vi "Shooter.vi"(4 "Ball Count":i8=3, 6 "Aquire Fail Action":T1, 7 "Distance":dbl, 8 "error in (no error)":errorcluster, 9 "Use Camera":bool, 10 "Test":bool, 11 "Fire":bool) -> (0 "error out":errorcluster, 3 "Shooter State":T1)   [LabVIEW 2011]
uses:
  ShooterStates.ctl
  Robot Global Data.vi
  <vilib>/Rock Robotics/WPI/Solenoid/Deprecated/WPI_SolenoidSetBool.vi
panel:
  in  "Second Spinup Timeout (ms)":u32=2000
  in  "PostSensor(ms)":u32=50
  in  "First Spinup Timeout (ms)":u32=3000
  out "Shot":bool
  in  "Top Rollers Speed":dbl=-1.0
  in  "Max Shoot Time (ms)":u32=2000
  # "Shoot"
  # "Spinup"
  # "Run Shooter\nOnly"
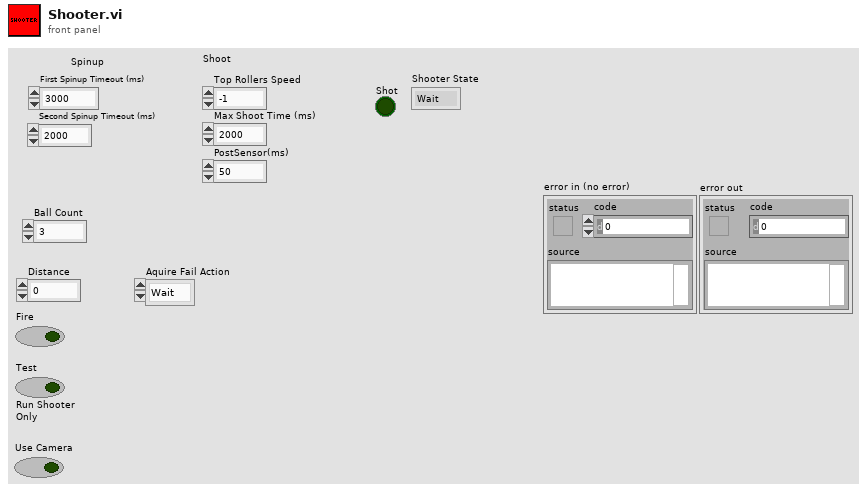
[diagram p1: front panel]
types:
  T1 = typedef "ShooterStates.ctl" = enum16{"Wait", "Aquire", "SpinUp", "Shoot", "Test"}
  T2 = typedef "Semaphore RefNum" = refnum<k1>
  T3 = cluster{"Aquire Target":bool, "Target Aquired":bool, "Attempts":dbl}
  T4 = typedef "ShooterData.ctl" = cluster{"Setpoint":dbl, "Speed":dbl, "Squish":dbl, "Shot Sensor":bool, "At Speed":bool}
  T5 = typedef "WPI_DigitalInputDevRef.ctl" = cluster{"DevStatus":errorcluster, "DIO Channel":T6, "Digital Module":T7}
  T6 = typedef "FPGA_DIOChannel.ctl" = enum8{"DIO 1", "DIO 2", "DIO 3", "DIO 4", "DIO 5", "DIO 6", "DIO 7", "DIO 8", "DIO 9", "DIO 10", "DIO 11", "DIO 12", "DIO 13", "DIO 14", "Invalid"}
  T7 = typedef "FPGA_TypedefDigitalModule.ctl" = enum16{"Digital Module 1", "Digital Module 2"}
  T8 = typedef "WPI_SolenoidDevRef.ctl" = cluster{"DevStatus":errorcluster, "Solenoid Module":T9, "Forward Solenoid Channel":T10, "Reverse Solenoid Channel":T10}
  T9 = typedef "FPGA_TypedefSolenoidModule.ctl" = enum16{"Solenoid Module 1", "Solenoid Module 2"}
  T10 = typedef "WPI_SolenoidChannel.ctl" = enum8{"Solenoid 1", "Solenoid 2", "Solenoid 3", "Solenoid 4", "Solenoid 5", "Solenoid 6", "Solenoid 7", "Solenoid 8", "Invalid"}
  T11 = typedef "WPI_MotorControlDeviceRef.ctl" = cluster{"DeviceStatus":errorcluster, "Type":enum16{"PWM", "CAN"}, "PWM":cluster{"Digital Module":T7, "PWM Channel":T12, "DeadBand":T13}, "CAN":cluster{"Device Number":u8, "Control Mode":T14, "Semaphore":T2, "Max Vout":dbl}, "Invert":bool, "TransformRef":T15, "InvTransformRef":T15}
  T12 = typedef "FPGA_DIOPWMChannel.ctl" = enum8{"PWM 1", "PWM 2", "PWM 3", "PWM 4", "PWM 5", "PWM 6", "PWM 7", "PWM 8", "PWM 9", "PWM 10", "Invalid"}
  T13 = typedef "WPI_PWMDeadband.ctl" = cluster{"Name":string, "maxPositivePwm":i32, "minPositivePwm":i32, "centerPwm":i32, "maxNegativePwm":i32, "minNegativePwm":i32, "angularRange":u16}
  T14 = typedef "WPI_CANJaguar_ControlMode.ctl" = enum8{"Percent VBus", "Current", "Speed", "Position", "Voltage"}
  T15 = typedef "WPI_PWMTransform_ConPane.ctl" = refnum<vi>
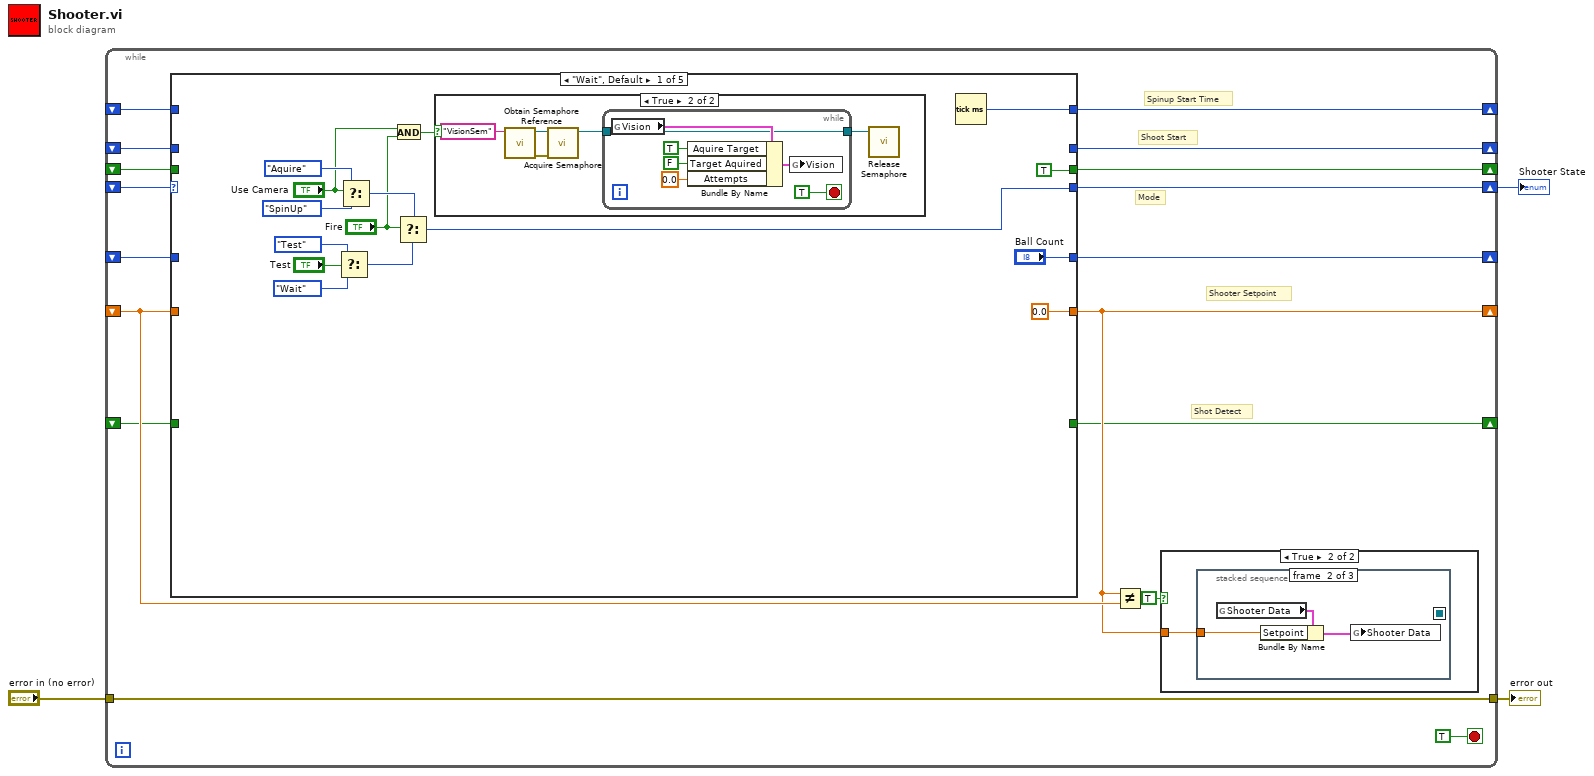
[diagram p0: block diagram]
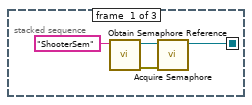
[diagram p3: hidden frame]
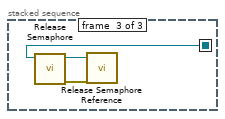
[diagram p4: hidden frame]
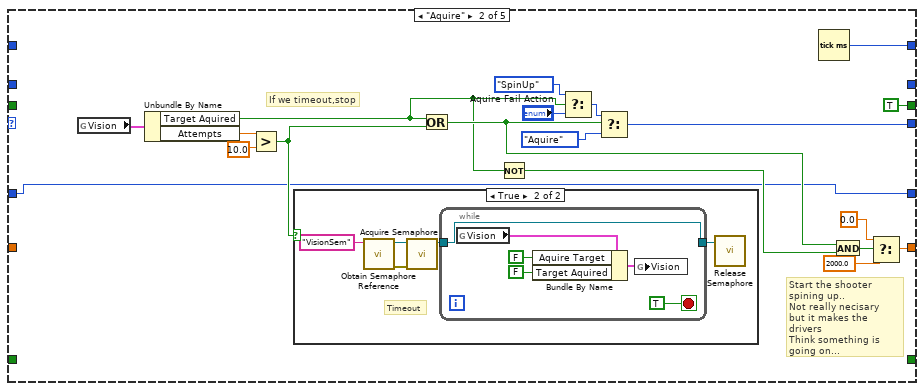
[diagram p6: hidden frame]
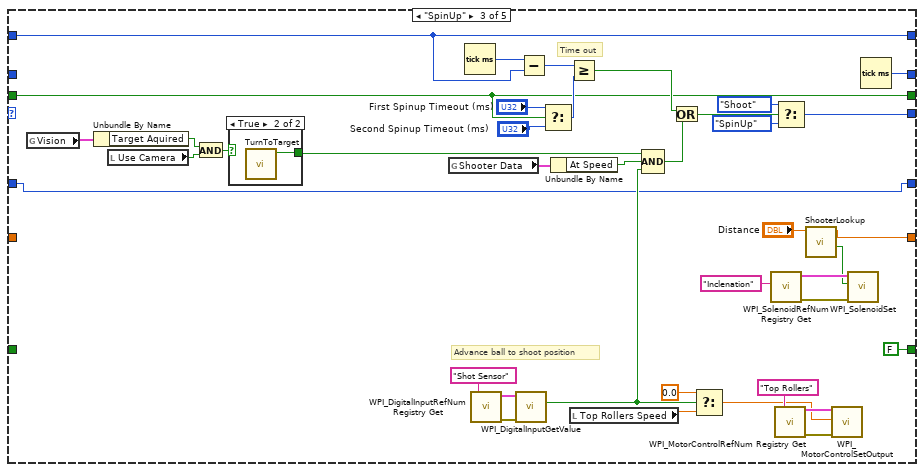
[diagram p8: hidden frame]
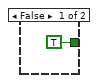
[diagram p9: hidden frame]
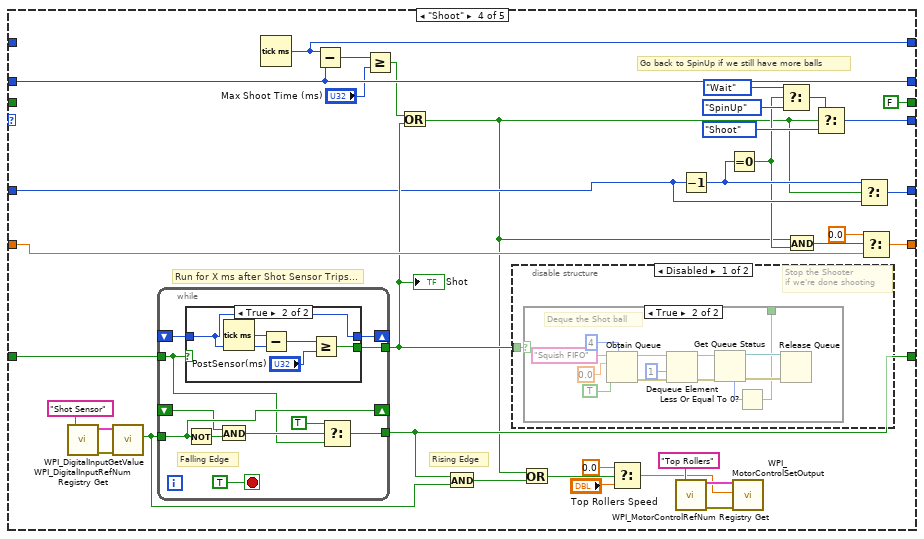
[diagram p10: hidden frame]
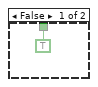
[diagram p11: hidden frame]
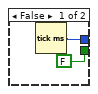
[diagram p13: hidden frame]
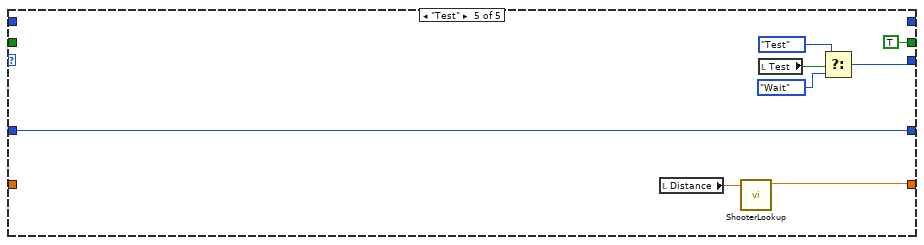
[diagram p14: hidden frame]
diagram:
  n1 = while {
    shift-right: [w12] -> _
    shift-left: _ -> [w13]
    shift-right: [w19] -> w3
    shift-left: _ -> [w20]
    shift-right: [w17] -> _
    shift-left: _ -> [w16]
    shift-right: [w15] -> _
    shift-left: _ -> [w14]
    shift-right: [w11] -> _
    shift-left: _ -> [w10]
    tunnel: "error in (no error)" -> [w9]
    tunnel: [w9] -> w1
    shift-right: [w6] -> _
    shift-left: _ -> [w7]
    shift-right: [w5] -> _
    shift-left: _ -> [w4]
    stop <- TRUE stop-if-true
    # "Shot Detect"
    # "Shooter Setpoint"
    # "Shoot Start"
    # "Spinup Start Time"
    # "Mode"
    n2 = case shown="\"Wait\", Default" w20 {
      tunnel: [w46 w74 w126 w163 w203] -> w19
      tunnel: [0.0 ("Output") w61 w96 w135 w201] -> w12
      tunnel: [_ _ w125 w162 _] -> w17
      tunnel: w13 -> [_ _ _ w151 _]
      tunnel: w16 -> [_ _ _ w162 _]
      tunnel: [w40 w72 w122 w147 _] -> w15
      tunnel: w14 -> [_ _ w122 _ _]
      tunnel: [_ _ FALSE w141 _] -> w11
      tunnel: w10 -> [_ _ _ w146 _]
      tunnel: w7 -> [_ _ w90 _ _]
      tunnel: [TRUE ("s") TRUE ("s") w90 FALSE ("s") TRUE ("s")] -> w6
      tunnel: ["Ball Count" w59 w89 w136 w198] -> w5
      tunnel: w4 -> [_ w59 w89 w134 w198]
      frame "Wait", Default {
        n3 = Select(t=ShooterStates."Test", s="Test", f=ShooterStates."Wait" ("Enum")) -> (s? t:f=w44:T1)
        n4 = Select(t=ShooterStates."Aquire", s="Use Camera", f=ShooterStates."SpinUp" ("Enum")) -> (s? t:f=w39:T1)
        n5 = And(x="Use Camera", y="Fire") -> (x .and. y?=w36:bool)
        n6 = Select(t=w39, s="Fire", f=w44) -> (s? t:f=w46:T1)
        n7 = case shown="True" w36 {
          frame False {
          }
          frame True {
            n8 = call <vilib>:"Obtain Semaphore Reference.vi"("name (unnamed)"="VisionSem") -> ("error out"=w50:errorcluster, "semaphore"=w51:T2)  [unwired: 4 in, 1 out]
            n9 = call <vilib>:"Acquire Semaphore.vi"("error in (no error)"=w50, "semaphore"=w51) -> ("semaphore out"=w48:T2)  [unwired: 3 in, 2 out]
            n10 = while {
              tunnel: w48 -> [w52]
              tunnel: [w52] -> w47
              stop <- TRUE stop-if-true
              n11 = global read "Robot Global Data.vi" "Vision"() -> (w57:T3)
              n12 = Bundle By Name(cluster=w57, "Aquire Target"=TRUE, "Target Aquired"=FALSE, "Attempts"=0.0) -> (w58:T3)
              n13 = global write "Robot Global Data.vi" "Vision"(w58) -> ()
            }
            n14 = call <vilib>:"Release Semaphore.vi"("semaphore"=w47) -> ()  [unwired: 5 in, 2 out]
          }
        }
        n15 = Tick Count (ms)() -> (millisecond timer value=w40:u32)
      }
      frame "Aquire" {
        # "Start the shooter\nspining up..\nNot really necisary \nbut it makes the drivers\nThink something is \ngoing on..."
        # "If we timeout,stop"
        n16 = global read "Robot Global Data.vi" "Vision"() -> (w77:T3)
        n17 = Unbundle By Name(w77) -> ("Target Aquired"=w64:bool, "Attempts"=w76:dbl)
        n18 = Greater?(x=w76, y=10.0) -> (0:w71:bool)
        n19 = case shown="True" w71 {
          frame False {
          }
          frame True {
            # "Timeout"
            n20 = call <vilib>:"Obtain Semaphore Reference.vi"("name (unnamed)"="VisionSem") -> ("error out"=w81:errorcluster, "semaphore"=w82:T2)  [unwired: 4 in, 1 out]
            n21 = call <vilib>:"Acquire Semaphore.vi"("error in (no error)"=w81, "semaphore"=w82) -> ("semaphore out"=w79:T2)  [unwired: 3 in, 2 out]
            n22 = while {
              tunnel: w79 -> [w83]
              tunnel: [w83] -> w78
              stop <- TRUE stop-if-true
              n23 = global read "Robot Global Data.vi" "Vision"() -> (w87:T3)
              n24 = Bundle By Name(cluster=w87, "Aquire Target"=FALSE, "Target Aquired"=FALSE) -> (w88:T3)
              n25 = global write "Robot Global Data.vi" "Vision"(w88) -> ()
            }
            n26 = call <vilib>:"Release Semaphore.vi"("semaphore"=w78) -> ()  [unwired: 5 in, 2 out]
          }
        }
        n27 = Or(x=w64, y=w71) -> (x .or. y?=w65:bool)
        n28 = Not(x=w64) -> (.not. x?=w63:bool)
        n29 = Select(t=ShooterStates."SpinUp" ("Enum"), s=w64, f="Aquire Fail Action") -> (s? t:f=w70:T1)
        n30 = Select(t=w70, s=w65, f=ShooterStates."Aquire" ("Enum")) -> (s? t:f=w74:T1)
        n31 = Tick Count (ms)() -> (millisecond timer value=w72:u32)
        n32 = And(x=w65, y=w63) -> (x .and. y?=w67:bool)
        n33 = Select(t=0.0 ("Speed"), s=w67, f=2000.0) -> (s? t:f=w61:dbl)
      }
      frame "SpinUp" {
        # "Advance ball to shoot position"
        # "Time out"
        n34 = global read "Robot Global Data.vi" "Vision"() -> (w116:T3)
        n35 = Unbundle By Name(w116) -> ("Target Aquired"=w114:bool)
        n36 = local read "Use Camera"() -> (w113:bool)
        n37 = And(x=w114, y=w113) -> (x .and. y?=w115:bool)
        n38 = case shown="True" w115 {
          tunnel: [TRUE ("On Target") w129] -> w99
          frame False {
          }
          frame True {
            n39 = call "TurnToTarget.vi"() -> ("On Target"=w129:bool)  [unwired: 11 in]
          }
        }
        n40 = global read "Robot Global Data.vi" "Shooter Data"() -> (w95:T4)
        n41 = Tick Count (ms)() -> (millisecond timer value=w124:u32)
        n42 = call <vilib>:"WPI_DigitalInputRefNum Registry Get.vi"("refnum name"="Shot Sensor") -> ("error out"=w107:errorcluster, "DigitalInputDevRef"=w106:T5)  [unwired: 9 in]
        n43 = call <vilib>:"WPI_DigitalInputGetValue.vi"("error in (no error)"=w107, "DigitalInputDevRef"=w106) -> ("Value"=w98:bool)  [unwired: 7 in, 2 out]
        n44 = Subtract(x=w124, y=w122) -> (x-y=w123:u32)
        n45 = Select(t="First Spinup Timeout (ms)", s=w90, f="Second Spinup Timeout (ms)") -> (s? t:f=w91:u32)
        n46 = Unbundle By Name(w95) -> ("At Speed"=w94:bool)
        n47 = Greater Or Equal?(x=w123, y=w91) -> (x >= y?=w111:bool)
        n48 = local read "Top Rollers Speed"() -> (w101:dbl)
        n49 = Compound Arithmetic op=AND(w99, w94, w98) -> (w97:bool)
        n50 = Or(x=w111, y=w97) -> (x .or. y?=w110:bool)
        n51 = Select(t=0.0, s=w98, f=w101) -> (s? t:f=w102:dbl)
        n52 = call <vilib>:"WPI_SolenoidRefNum Registry Get.vi"("refnum name"="Inclenation") -> ("error out"=w121:errorcluster, "SolenoidDevRef"=w120:T8)  [unwired: 9 in]
        n53 = call <vilib>:"WPI_MotorControlRefNum Registry Get.vi"("refnum name"="Top Rollers") -> ("error out"=w104:errorcluster, "MotorControlDevRef"=w103:T11)  [unwired: 9 in]
        n54 = Select(t=ShooterStates."Shoot" ("Enum"), s=w110, f=ShooterStates."SpinUp" ("Enum")) -> (s? t:f=w126:T1)
        n55 = call "ShooterLookup.vi"("Distance"="Distance") -> ("Elevation"=w118:bool, "Speed"=w96:dbl)  [unwired: 9 in]
        n56 = call <vilib>:"WPI_MotorControlSetOutput.vi"("error in (no error)"=w104, "Output"=w102, "MotorControlDevRef"=w103) -> ()  [unwired: 7 in, 2 out]
        n57 = call-poly <vilib>:"WPI_SolenoidSet.vi"("error in (no error)"=w121, "Value"=w118, "SolenoidDevRef"=w120) -> ()  [unwired: 7 in, 2 out]
        n58 = Tick Count (ms)() -> (millisecond timer value=w125:u32)
      }
      frame "Shoot" {
        # "Rising Edge"
        # "Go back to SpinUp if we still have more balls"
        # "Run for X ms after Shot Sensor Trips..."
        n59 = call <vilib>:"WPI_DigitalInputRefNum Registry Get.vi"("refnum name"="Shot Sensor") -> ("error out"=w149:errorcluster, "DigitalInputDevRef"=w148:T5)  [unwired: 9 in]
        n60 = call <vilib>:"WPI_DigitalInputGetValue.vi"("error in (no error)"=w149, "DigitalInputDevRef"=w148) -> ("Value"=w140:bool)  [unwired: 7 in, 2 out]
        n61 = while {
          tunnel: w140 -> [w189]
          shift-right: [w189] -> _
          shift-left: _ -> [w187]
          tunnel: w146 -> [w181]
          shift-right: [w186] -> _
          shift-left: _ -> [w185]
          tunnel: [w182] -> w141
          tunnel: [w180] -> w142
          stop <- TRUE stop-if-true
          # "Falling Edge"
          n62 = case shown="True" w181 {
            tunnel: [w192 w194] -> w186
            tunnel: w185 -> [_ w194]
            tunnel: [FALSE w193] -> w180
            frame False {
              n63 = Tick Count (ms)() -> (millisecond timer value=w192:u32)
            }
            frame True {
              n64 = Tick Count (ms)() -> (millisecond timer value=w196:u32)
              n65 = Subtract(x=w196, y=w194) -> (x-y=w197:u32)
              n66 = Greater Or Equal?(x=w197, y="PostSensor(ms)") -> (x >= y?=w193:bool)
            }
          }
          n67 = Not(x=w189) -> (.not. x?=w188:bool)
          n68 = And(x=w187, y=w188) -> (x .and. y?=w183:bool)
          n69 = Select(t=TRUE, s=w183, f=w181) -> (s? t:f=w182:bool)
        }
        "Shot" <- w142
        n70 = Tick Count (ms)() -> (millisecond timer value=w147:u32)
        n71 = Subtract(x=w147, y=w162) -> (x-y=w161:u32)
        n72 = Greater Or Equal?(x=w161, y="Max Shoot Time (ms)") -> (x >= y?=w154:bool)
        n73 = Or(x=w154, y=w142) -> (x .or. y?=w130:bool)
        n74 = And(x=w141, y=w140) -> (x .and. y?=w138:bool)
        n75 = disable-structure shown="Disabled" {
          disable-tunnel: w142 -> [w165 _]
          frame Disabled {
            # "Stop the Shooter\nif we're done shooting"
            n76 = case shown="True" w165 {
              tunnel: [TRUE w167] -> _
              frame False {
              }
              frame True {
                # "Deque the Shot ball"
                n77 = Obtain Queue(max queue size (-1, unlimited)=4, name (unnamed)="Squish FIFO", element data type=sgl 0.0 ("Voltage"), create if not found? (T)=TRUE) -> (queue out=w176:refnum<queue>, error out=w177:errorcluster)  [unwired: 1 in, 1 out]
                n78 = Dequeue Element(queue=w176, timeout in ms (-1)=1, error in (no error)=w177) -> (queue out=w172:refnum<queue>, error out=w171:errorcluster)  [unwired: 2 out]
                n79 = Get Queue Status(queue=w172, error in (no error)=w171) -> (queue out=w170:refnum<queue>, error out=w169:errorcluster, # elements in queue=w168:i32)  [unwired: 1 in, 5 out]
                n80 = Less Or Equal To 0?(x=w168) -> (x <= 0?=w167:bool)
                n81 = Release Queue(queue=w170, error in (no error)=w169) -> ()  [unwired: 1 in, 3 out]
              }
            }
          }
          frame Enabled {
          }
        }
        n82 = Or(x=w130, y=w138) -> (x .or. y?=w139:bool)
        n83 = Select(t=0.0 ("f"), s=w139, f="Top Rollers Speed") -> (s? t:f=w156:dbl)
        n84 = call <vilib>:"WPI_MotorControlRefNum Registry Get.vi"("refnum name"="Top Rollers") -> ("error out"=w158:errorcluster, "MotorControlDevRef"=w157:T11)  [unwired: 9 in]
        n85 = Decrement(x=w134) -> (x-1=w132:i8)
        n86 = Equal To 0?(x=w132) -> (x = 0?=w131:bool)
        n87 = call <vilib>:"WPI_MotorControlSetOutput.vi"("error in (no error)"=w158, "Output"=w156, "MotorControlDevRef"=w157) -> ()  [unwired: 7 in, 2 out]
        n88 = Select(t=ShooterStates."Wait" ("Enum"), s=w131, f=ShooterStates."SpinUp" ("Enum")) -> (s? t:f=w145:T1)
        n89 = And(x=w130, y=w131) -> (x .and. y?=w133:bool)
        n90 = Select(t=w145, s=w130, f=ShooterStates."Shoot" ("Enum")) -> (s? t:f=w163:T1)
        n91 = Select(t=w132, s=w130, f=w134) -> (s? t:f=w136:i8)
        n92 = Select(t=0.0, s=w133, f=w151) -> (s? t:f=w135:dbl)
      }
      frame "Test" {
        n93 = local read "Distance"() -> (w200:dbl)
        n94 = call "ShooterLookup.vi"("Distance"=w200) -> ("Speed"=w201:dbl)  [unwired: 9 in, 1 out]
        n95 = local read "Test"() -> (w202:bool)
        n96 = Select(t=ShooterStates."Test", s=w202, f=ShooterStates."Wait" ("Enum")) -> (s? t:f=w203:T1)
      }
    }
    n97 = Not Equal?(x=w12, y=w13) -> ()  [unwired: 1 out]
    n98 = case shown="True" TRUE {
      tunnel: w12 -> [_ w21]
      frame False {
      }
      frame True {
        n99 = stacked-sequence {
          seq-local: [w22 _ _] -> [_ _ w29]
          tunnel: w21 -> [_ w26 _]
          frame #0 {
            n100 = call <vilib>:"Obtain Semaphore Reference.vi"("name (unnamed)"="ShooterSem") -> ("error out"=w24:errorcluster, "semaphore"=w25:T2)  [unwired: 4 in, 1 out]
            n101 = call <vilib>:"Acquire Semaphore.vi"("error in (no error)"=w24, "semaphore"=w25) -> ("semaphore out"=w22:T2)  [unwired: 3 in, 2 out]
          }
          frame #1 {
            n102 = global read "Robot Global Data.vi" "Shooter Data"() -> (w27:T4)
            n103 = Bundle By Name(cluster=w27, "Setpoint"=w26) -> (w28:T4)
            n104 = global write "Robot Global Data.vi" "Shooter Data"(w28) -> ()
          }
          frame #2 {
            n105 = call <vilib>:"Release Semaphore.vi"("semaphore"=w29) -> ("error out"=w31:errorcluster, "semaphore out"=w30:T2)  [unwired: 5 in]
            n106 = call <vilib>:"Release Semaphore Reference.vi"("error in (no error)"=w31, "semaphore"=w30) -> ()  [unwired: 8 in, 2 out]
          }
        }
      }
    }
  }
  "Shooter State" <- w3
  "error out" <- w1
